vi "Get Measurements P2.vi"(0 "Image In":T1, 11 "Error In":errorcluster) -> (4 "Image Out":T1, 12 "Calibrated Results (P2 Hole)":sgl format="%.2f", 13 "Calibrated Results (P2 Right Edge Angle)":sgl, 14 "Calibrated Results (P2 Left Edge Angles)":sgl, 15 "Error Out":errorcluster)   [LabVIEW 2020]
uses:
  <vilib>/vision/Image Controls.llb/IMAQ Image.ctl
  <vilib>/vision/Measure.llb/Edge Options.ctl
  <vilib>/vision/Measure.llb/Edge Polarity.ctl
  <vilib>/vision/Measure.llb/Straight Edge Options.ctl
  <vilib>/vision/Measure.llb/Straight Edge Process.ctl
  <vilib>/vision/NI_Vision_Development_Module.lvlib
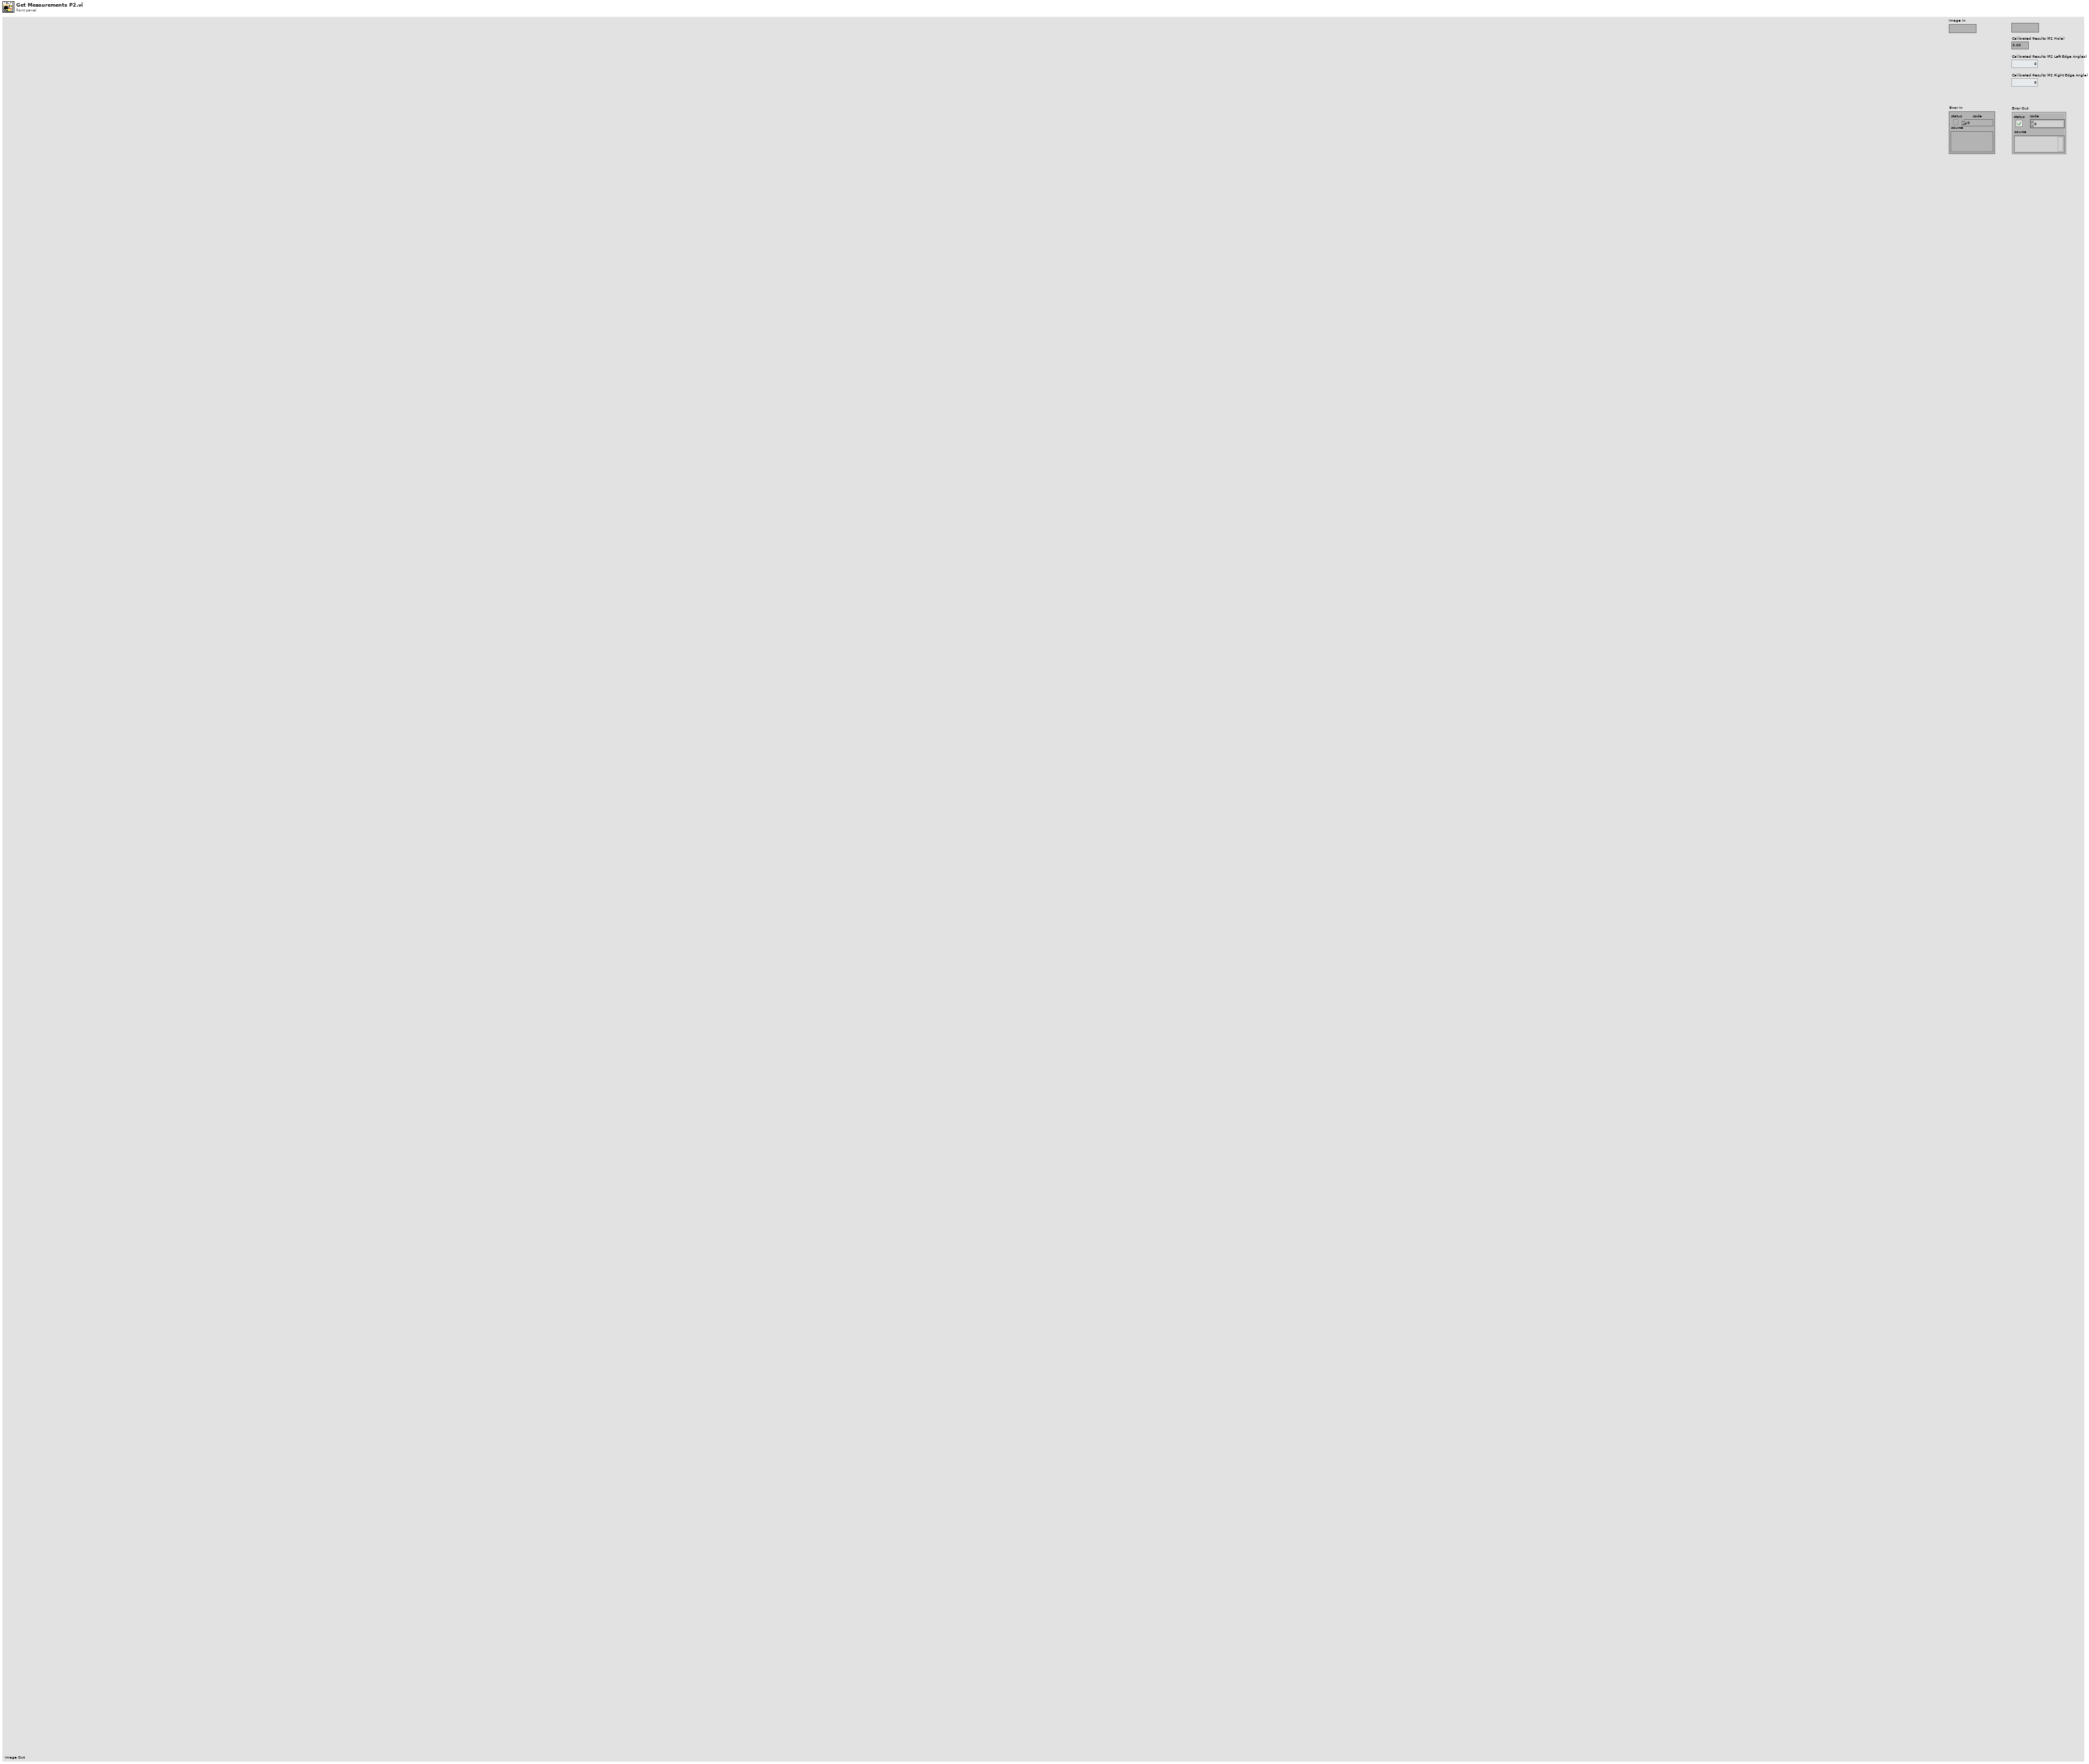
[diagram p1: front panel]
types:
  T1 = typedef "IMAQ Image.ctl" = refnum<image>
  T2 = cluster{"Feature":u32, "Points IDs":cluster{"GUID":string, "Index":i32}[]}[]
  T3 = typedef "Edge Options.ctl" = cluster{"Edge Polarity":T4, "Kernel Size":u32, "Width":u32, "Minimum Edge Strength":sgl, "Interpolation Type":enum32{"Zero Order", "Bilinear", "Quadratic", "Cubic", "Bilinear Fixed"}, "Data Processing Method":enum32{"Average", "Median"}}
  T4 = typedef "Edge Polarity.ctl" = u32
  T5 = cluster{"Search Direction":u32, "Edge Options":T3, "Show Search Area":bool, "Show Search Lines":bool, "Show Edges Found":bool, "Show Result":bool, "Search Area Color":u32, "Search Lines Color":u32, "Edge Locations Color":u32, "Result Color":u32, "Overlay Group Name":string}
  T6 = typedef "Straight Edge Options.ctl" = cluster{"Number of Lines":i32, "Type":T7, "Min. Score":dbl, "Max. Score":dbl, "Orientation":dbl, "Angle Range":dbl, "Angle Tolerance":dbl, "Step Size":u32, "Min. SNR (db)":dbl, "Min. Points (%)":dbl, "Hough Iterations":i32}
  T7 = typedef "Straight Edge Process.ctl" = enum32{"First Edge Rake", "Best Edge Rake", "Hough Edge Rake", "First Edge Projection", "Best Edge Projection"}
  T8 = cluster{"Global Rectangle":i32[], "Contours":cluster{"ID":enum32{"External", "Internal"}, "Type":u32, "Coordinates":i32[]}[]}
  T9 = cluster{"Origin":cluster{"X":sgl, "Y":sgl}, "Angle (deg)":sgl, "Axis Reference":u32}
  T10 = enum16{"Reset", "Update Coordinate System", "Get Coordinate System"}
  T11 = cluster{"Search  Direction":u32, "Edge Options":T3, "Show Search Area":bool, "Show Search Lines":bool, "Show Edges Found":bool, "Show Result":bool, "Search Area Color":u32, "Search Lines Color":u32, "Edge Locations Color":u32, "Result Color":u32, "Overlay Group Name":string}
  T12 = cluster{"Process":enum16{"Get First Edge", "Get First + Last Edge", "Get All Edges", "Get Best Edge"}, "Step Size":i32, "Max Pixel Radius":i32}
  T13 = typedef "IMAQ Coordinate System" = cluster{"Reference System":cluster{"Origin":cluster{"X":sgl, "Y":sgl}, "Angle (deg)":sgl, "Axis Reference":u32}, "Measurement System":cluster{"Origin":cluster{"X":sgl, "Y":sgl}, "Angle (deg)":sgl, "Axis Reference":u32}}
  T14 = typedef "ROI Descriptor" = cluster{"Global Rectangle":i32[], "Contours":cluster{"ID":enum32{"External", "Internal"}, "Type":u32, "Coordinates":i32[]}[]}
  T15 = cluster{"Point1 (Pixels)":cluster{"X":sgl, "Y":sgl}, "Point2 (Pixels)":cluster{"X":sgl, "Y":sgl}, "Point1 (Real-World)":cluster{"X":sgl, "Y":sgl}, "Point2 (Real-World)":cluster{"X":sgl, "Y":sgl}, "Angle (Pixel)":dbl, "Angle (Real-World)":dbl, "Score":dbl, "Straightness":dbl, "Average SNR (db)":dbl, "Calibration Valid":bool}[]
  T16 = cluster{"Point1 (Pixels)":cluster{"X":sgl, "Y":sgl}, "Point2 (Pixels)":cluster{"X":sgl, "Y":sgl}, "Point1 (Real-World)":cluster{"X":sgl, "Y":sgl}, "Point2 (Real-World)":cluster{"X":sgl, "Y":sgl}, "Angle (Pixel)":dbl, "Angle (Real-World)":dbl, "Score":dbl, "Straightness":dbl, "Average SNR (db)":dbl, "Calibration Valid":bool}
  T17 = cluster{"Center (Pixels)":cluster{"X":sgl, "Y":sgl}, "Radius (Pixels)":dbl, "Center (Real-World)":cluster{"X":sgl, "Y":sgl}, "Radius (Real-World)":dbl, "Roundness (Real-World)":dbl, "Average Strength":dbl, "Average SNR (dB)":dbl}
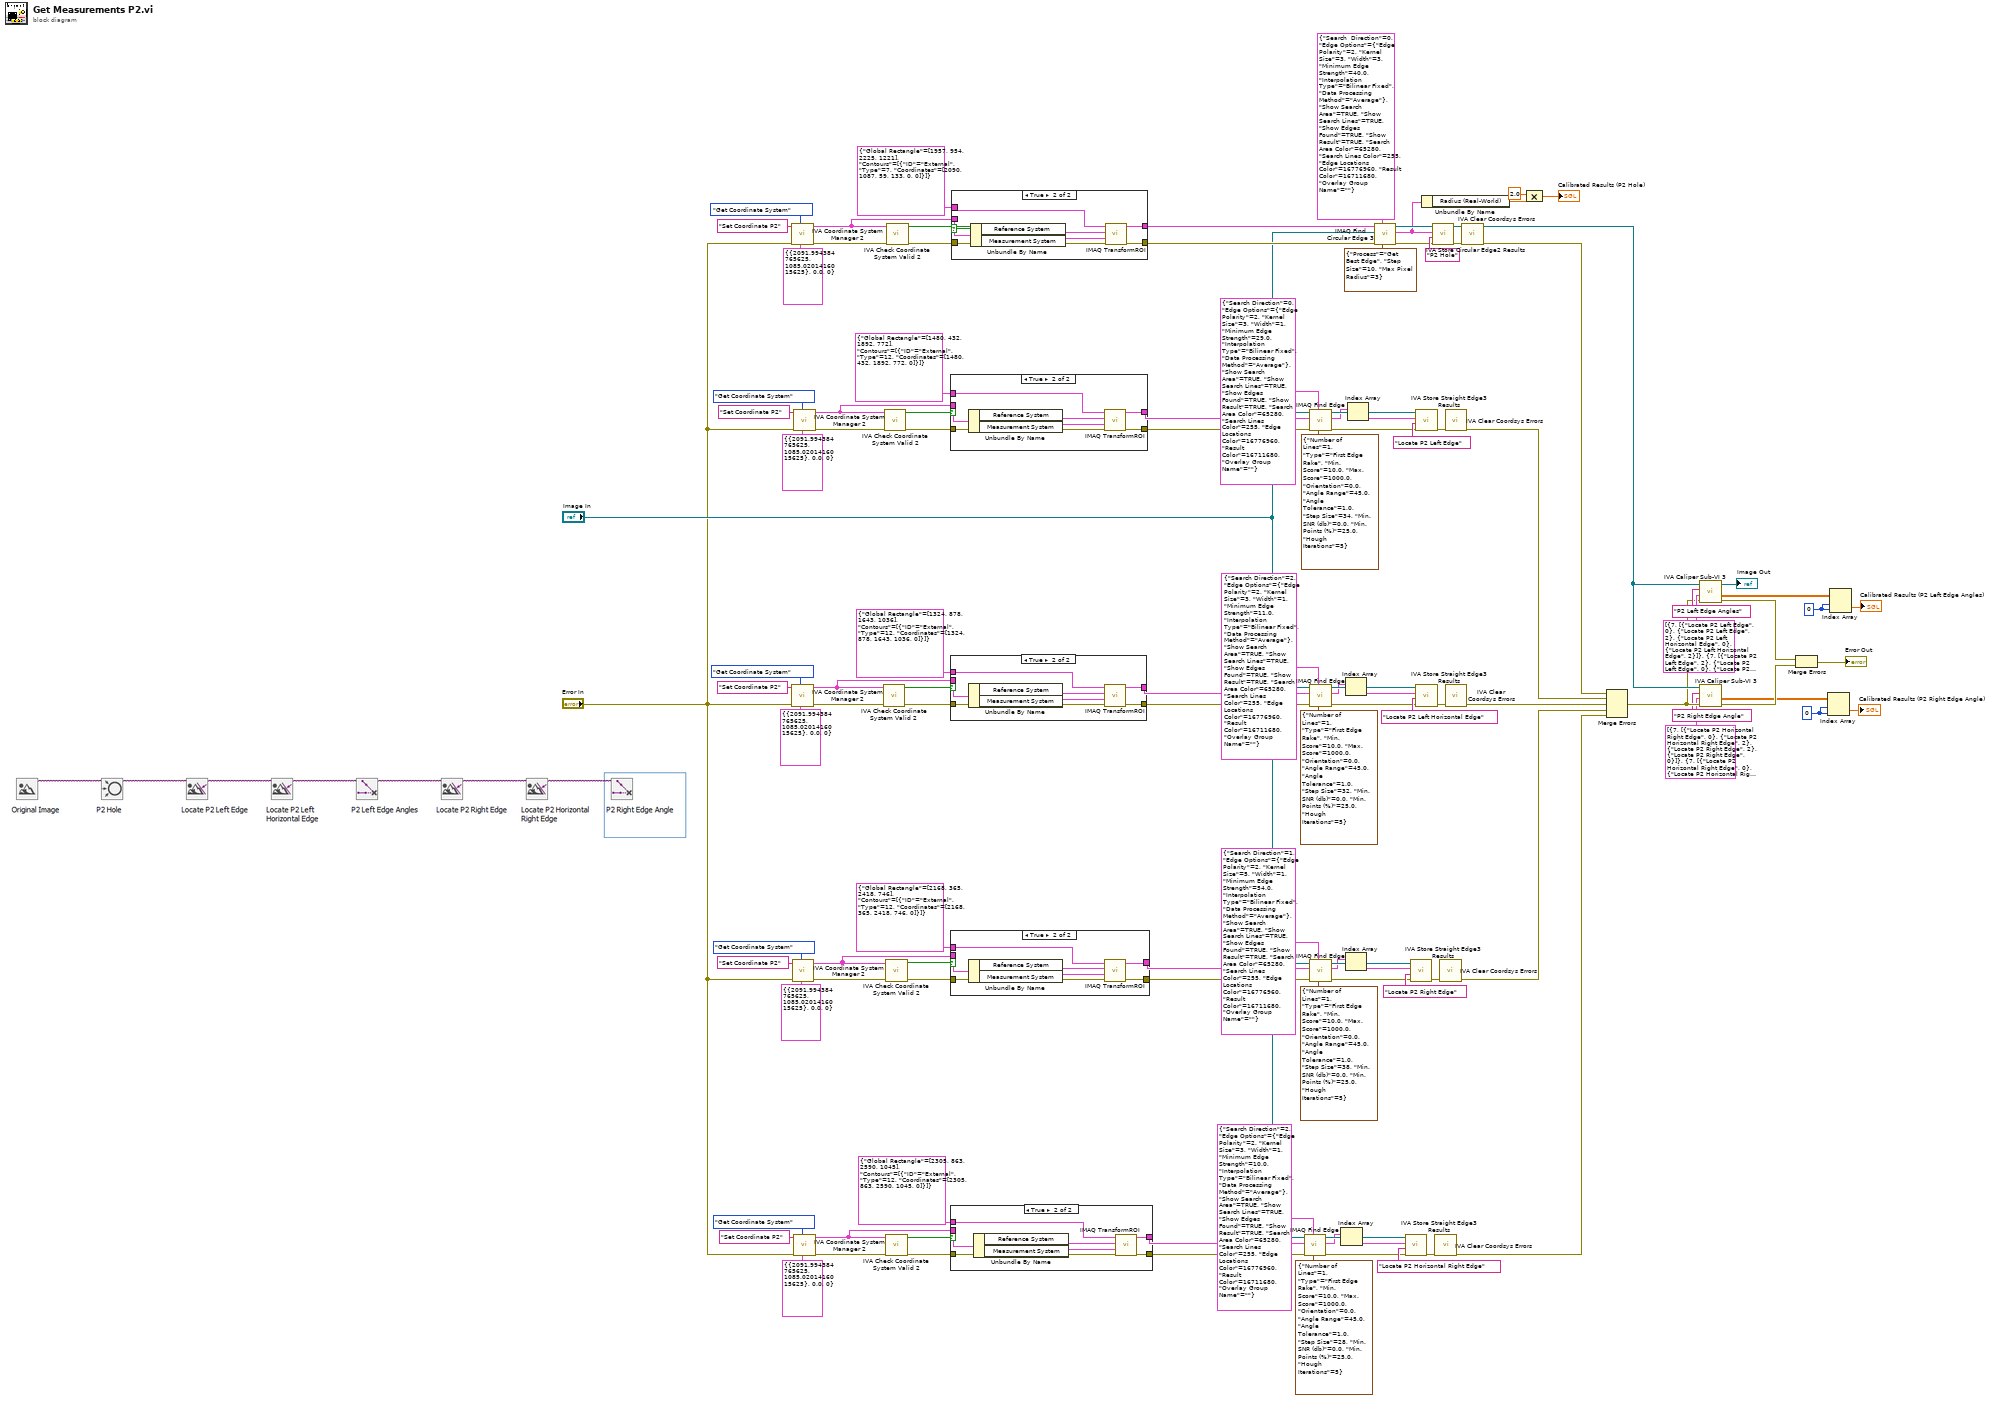
[diagram p0: block diagram]
diagram:
  w5 = 0 ("disabled index (col)")
  w6 = 0 ("disabled index (col)")
  n1 = call <vilib>:"IVA Coordinate System Manager 2.vi"("Reference System"=T9 {"Origin"={"X"=2091.9944, "Y"=1085.0201}, "Angle (deg)"=0.0, "Axis Reference"=0}, "Function"=T10."Get Coordinate System", "error in (no error)"="Error In", "Coordinate System Name"="Set Coordinate P2") -> ("error out"=w109:errorcluster, "Coordinate System Out"=w111:T13)  [unwired: 3 in, 3 out]
  n2 = call <vilib>:"IVA Coordinate System Manager 2.vi"("Reference System"=T9 {"Origin"={"X"=2091.9944, "Y"=1085.0201}, "Angle (deg)"=0.0, "Axis Reference"=0}, "Function"=T10."Get Coordinate System", "error in (no error)"="Error In", "Coordinate System Name"="Set Coordinate P2") -> ("error out"=w75:errorcluster, "Coordinate System Out"=w77:T13)  [unwired: 3 in, 3 out]
  n3 = call <vilib>:"IVA Coordinate System Manager 2.vi"("Reference System"=T9 {"Origin"={"X"=2091.9944, "Y"=1085.0201}, "Angle (deg)"=0.0, "Axis Reference"=0}, "Function"=T10."Get Coordinate System", "error in (no error)"="Error In", "Coordinate System Name"="Set Coordinate P2") -> ("error out"=w57:errorcluster, "Coordinate System Out"=w59:T13)  [unwired: 3 in, 3 out]
  n4 = call <vilib>:"IVA Coordinate System Manager 2.vi"("Reference System"=T9 {"Origin"={"X"=2091.9944, "Y"=1085.0201}, "Angle (deg)"=0.0, "Axis Reference"=0}, "Function"=T10."Get Coordinate System", "error in (no error)"="Error In", "Coordinate System Name"="Set Coordinate P2") -> ("error out"=w93:errorcluster, "Coordinate System Out"=w95:T13)  [unwired: 3 in, 3 out]
  n5 = call <vilib>:"IVA Coordinate System Manager 2.vi"("Reference System"=T9 {"Origin"={"X"=2091.9944, "Y"=1085.0201}, "Angle (deg)"=0.0, "Axis Reference"=0}, "Function"=T10."Get Coordinate System", "error in (no error)"="Error In", "Coordinate System Name"="Set Coordinate P2") -> ("error out"=w39:errorcluster, "Coordinate System Out"=w41:T13)  [unwired: 3 in, 3 out]
  n6 = call <vilib>:"IVA Check Coordinate System Valid 2.vi"("error in (no error)"=w75, "Coordinate System"=w77) -> ("error out"=w74:errorcluster, "Valid?"=w76:bool)  [unwired: 8 out]
  n7 = call <vilib>:"IVA Check Coordinate System Valid 2.vi"("error in (no error)"=w93, "Coordinate System"=w95) -> ("error out"=w92:errorcluster, "Valid?"=w94:bool)  [unwired: 8 out]
  n8 = call <vilib>:"IVA Check Coordinate System Valid 2.vi"("error in (no error)"=w57, "Coordinate System"=w59) -> ("error out"=w56:errorcluster, "Valid?"=w58:bool)  [unwired: 8 out]
  n9 = call <vilib>:"IVA Check Coordinate System Valid 2.vi"("error in (no error)"=w39, "Coordinate System"=w41) -> ("error out"=w38:errorcluster, "Valid?"=w40:bool)  [unwired: 8 out]
  n10 = call <vilib>:"IVA Check Coordinate System Valid 2.vi"("error in (no error)"=w109, "Coordinate System"=w111) -> ("error out"=w108:errorcluster, "Valid?"=w110:bool)  [unwired: 8 out]
  n11 = case shown="True" w94 {
    tunnel: T8 {"Global Rectangle"=[1480, 432, 1892, 772], "Contours"=[{"ID"=enum."External", "Type"=12, "Coordinates"=[1480, 432, 1892, 772, 0]}]} ("ROI Descriptor") -> [w117 w124]
    tunnel: [w117 w121] -> w91
    tunnel: [w116 w120] -> w89
    tunnel: w95 -> [_ w119]
    tunnel: w92 -> [w116 w118]
    frame False {
    }
    frame True {
      n12 = Unbundle By Name(w119) -> ("Reference System"=w123:T9, "Measurement System"=w122:T9)
      n13 = call "IMAQ TransformROI"("error in (no error)"=w118, "New Reference"=w122, "Base Reference"=w123, "ROI Descriptor"=w124) -> ("error out"=w120:errorcluster, "ROI Descriptor out"=w121:T14)  [unwired: 6 out]
    }
  }
  n14 = case shown="True" w76 {
    tunnel: T8 {"Global Rectangle"=[1324, 878, 1643, 1036], "Contours"=[{"ID"=enum."External", "Type"=12, "Coordinates"=[1324, 878, 1643, 1036, 0]}]} ("ROI Descriptor") -> [w126 w133]
    tunnel: [w126 w130] -> w73
    tunnel: [w125 w129] -> w71
    tunnel: w77 -> [_ w128]
    tunnel: w74 -> [w125 w127]
    frame False {
    }
    frame True {
      n15 = Unbundle By Name(w128) -> ("Reference System"=w132:T9, "Measurement System"=w131:T9)
      n16 = call "IMAQ TransformROI"("error in (no error)"=w127, "New Reference"=w131, "Base Reference"=w132, "ROI Descriptor"=w133) -> ("error out"=w129:errorcluster, "ROI Descriptor out"=w130:T14)  [unwired: 6 out]
    }
  }
  n17 = case shown="True" w58 {
    tunnel: T8 {"Global Rectangle"=[2168, 365, 2418, 746], "Contours"=[{"ID"=enum."External", "Type"=12, "Coordinates"=[2168, 365, 2418, 746, 0]}]} ("ROI Descriptor") -> [w135 w142]
    tunnel: [w135 w139] -> w55
    tunnel: [w134 w138] -> w53
    tunnel: w59 -> [_ w137]
    tunnel: w56 -> [w134 w136]
    frame False {
    }
    frame True {
      n18 = Unbundle By Name(w137) -> ("Reference System"=w141:T9, "Measurement System"=w140:T9)
      n19 = call "IMAQ TransformROI"("error in (no error)"=w136, "New Reference"=w140, "Base Reference"=w141, "ROI Descriptor"=w142) -> ("error out"=w138:errorcluster, "ROI Descriptor out"=w139:T14)  [unwired: 6 out]
    }
  }
  n20 = case shown="True" w40 {
    tunnel: T8 {"Global Rectangle"=[2305, 863, 2590, 1045], "Contours"=[{"ID"=enum."External", "Type"=12, "Coordinates"=[2305, 863, 2590, 1045, 0]}]} ("ROI Descriptor") -> [w144 w151]
    tunnel: [w144 w148] -> w37
    tunnel: [w143 w147] -> w35
    tunnel: w41 -> [_ w146]
    tunnel: w38 -> [w143 w145]
    frame False {
    }
    frame True {
      n21 = Unbundle By Name(w146) -> ("Reference System"=w150:T9, "Measurement System"=w149:T9)
      n22 = call "IMAQ TransformROI"("error in (no error)"=w145, "New Reference"=w149, "Base Reference"=w150, "ROI Descriptor"=w151) -> ("error out"=w147:errorcluster, "ROI Descriptor out"=w148:T14)  [unwired: 6 out]
    }
  }
  n23 = case shown="True" w110 {
    tunnel: T8 {"Global Rectangle"=[1957, 954, 2225, 1221], "Contours"=[{"ID"=enum."External", "Type"=7, "Coordinates"=[2090, 1087, 59, 133, 0, 0]}]} ("ROI Descriptor") -> [w153 w160]
    tunnel: [w153 w157] -> w106
    tunnel: [w152 w156] -> w105
    tunnel: w111 -> [_ w155]
    tunnel: w108 -> [w152 w154]
    frame False {
    }
    frame True {
      n24 = Unbundle By Name(w155) -> ("Reference System"=w159:T9, "Measurement System"=w158:T9)
      n25 = call "IMAQ TransformROI"("error in (no error)"=w154, "New Reference"=w158, "Base Reference"=w159, "ROI Descriptor"=w160) -> ("error out"=w156:errorcluster, "ROI Descriptor out"=w157:T14)  [unwired: 6 out]
    }
  }
  n26 = call "IMAQ Find Edge"("Line Fit Options"=T6 {"Number of Lines"=1, "Type"=enum."First Edge Rake", "Min. Score"=10.0, "Max. Score"=1000.0, "Orientation"=0.0, "Angle Range"=45.0, "Angle Tolerance"=1.0, "Step Size"=28, "Min. SNR (db)"=0.0, "Min. Points (%)"=25.0, "Hough Iterations"=5} ("Fit Options"), "Options"=T5 {"Search Direction"=2, "Edge Options"={"Edge Polarity"=2, "Kernel Size"=3, "Width"=1, "Minimum Edge Strength"=10.0, "Interpolation Type"=enum."Bilinear Fixed", "Data Processing Method"=enum."Average"}, "Show Search Area"=TRUE, "Show Search Lines"=TRUE, "Show Edges Found"=TRUE, "Show Result"=TRUE, "Search Area Color"=65280, "Search Lines Color"=255, "Edge Locations Color"=16776960, "Result Color"=16711680, "Overlay Group Name"=""}, "error in (no error)"=w35, "ROI Descriptor"=w37, "Image"="Image In") -> ("error out"=w30:errorcluster, "Straight Edges"=w29:T15, "Image Out"=w31:T1)  [unwired: 1 in, 3 out]
  n27 = call "IMAQ Find Edge"("Line Fit Options"=T6 {"Number of Lines"=1, "Type"=enum."First Edge Rake", "Min. Score"=10.0, "Max. Score"=1000.0, "Orientation"=0.0, "Angle Range"=45.0, "Angle Tolerance"=1.0, "Step Size"=34, "Min. SNR (db)"=0.0, "Min. Points (%)"=25.0, "Hough Iterations"=5} ("Fit Options"), "Options"=T5 {"Search Direction"=0, "Edge Options"={"Edge Polarity"=2, "Kernel Size"=3, "Width"=1, "Minimum Edge Strength"=29.0, "Interpolation Type"=enum."Bilinear Fixed", "Data Processing Method"=enum."Average"}, "Show Search Area"=TRUE, "Show Search Lines"=TRUE, "Show Edges Found"=TRUE, "Show Result"=TRUE, "Search Area Color"=65280, "Search Lines Color"=255, "Edge Locations Color"=16776960, "Result Color"=16711680, "Overlay Group Name"=""}, "error in (no error)"=w89, "ROI Descriptor"=w91, "Image"="Image In") -> ("error out"=w84:errorcluster, "Straight Edges"=w83:T15, "Image Out"=w85:T1)  [unwired: 1 in, 3 out]
  n28 = call "IMAQ Find Edge"("Line Fit Options"=T6 {"Number of Lines"=1, "Type"=enum."First Edge Rake", "Min. Score"=10.0, "Max. Score"=1000.0, "Orientation"=0.0, "Angle Range"=45.0, "Angle Tolerance"=1.0, "Step Size"=32, "Min. SNR (db)"=0.0, "Min. Points (%)"=25.0, "Hough Iterations"=5} ("Fit Options"), "Options"=T5 {"Search Direction"=2, "Edge Options"={"Edge Polarity"=2, "Kernel Size"=3, "Width"=1, "Minimum Edge Strength"=11.0, "Interpolation Type"=enum."Bilinear Fixed", "Data Processing Method"=enum."Average"}, "Show Search Area"=TRUE, "Show Search Lines"=TRUE, "Show Edges Found"=TRUE, "Show Result"=TRUE, "Search Area Color"=65280, "Search Lines Color"=255, "Edge Locations Color"=16776960, "Result Color"=16711680, "Overlay Group Name"=""}, "error in (no error)"=w71, "ROI Descriptor"=w73, "Image"="Image In") -> ("error out"=w66:errorcluster, "Straight Edges"=w65:T15, "Image Out"=w67:T1)  [unwired: 1 in, 3 out]
  n29 = call "IMAQ Find Edge"("Line Fit Options"=T6 {"Number of Lines"=1, "Type"=enum."First Edge Rake", "Min. Score"=10.0, "Max. Score"=1000.0, "Orientation"=0.0, "Angle Range"=45.0, "Angle Tolerance"=1.0, "Step Size"=38, "Min. SNR (db)"=0.0, "Min. Points (%)"=25.0, "Hough Iterations"=5} ("Fit Options"), "Options"=T5 {"Search Direction"=1, "Edge Options"={"Edge Polarity"=2, "Kernel Size"=5, "Width"=1, "Minimum Edge Strength"=54.0, "Interpolation Type"=enum."Bilinear Fixed", "Data Processing Method"=enum."Average"}, "Show Search Area"=TRUE, "Show Search Lines"=TRUE, "Show Edges Found"=TRUE, "Show Result"=TRUE, "Search Area Color"=65280, "Search Lines Color"=255, "Edge Locations Color"=16776960, "Result Color"=16711680, "Overlay Group Name"=""}, "error in (no error)"=w53, "ROI Descriptor"=w55, "Image"="Image In") -> ("error out"=w48:errorcluster, "Straight Edges"=w47:T15, "Image Out"=w49:T1)  [unwired: 1 in, 3 out]
  n30 = Index Array(array=w29) -> (element=w32:T16)  [unwired: 1 in]
  n31 = Index Array(array=w65) -> (element=w68:T16)  [unwired: 1 in]
  n32 = Index Array(array=w47) -> (element=w50:T16)  [unwired: 1 in]
  n33 = Index Array(array=w83) -> (element=w86:T16)  [unwired: 1 in]
  n34 = call "IMAQ Find Circular Edge 3"("Circle Fit Options"=T12 {"Process"=enum."Get Best Edge", "Step Size"=10, "Max Pixel Radius"=3}, "Options"=T11 {"Search  Direction"=0, "Edge Options"={"Edge Polarity"=2, "Kernel Size"=3, "Width"=3, "Minimum Edge Strength"=40.0, "Interpolation Type"=enum."Bilinear Fixed", "Data Processing Method"=enum."Average"}, "Show Search Area"=TRUE, "Show Search Lines"=TRUE, "Show Edges Found"=TRUE, "Show Result"=TRUE, "Search Area Color"=65280, "Search Lines Color"=255, "Edge Locations Color"=16776960, "Result Color"=16711680, "Overlay Group Name"=""}, "error in (no error)"=w105, "ROI Descriptor"=w106, "Image"="Image In") -> ("error out"=w102:errorcluster, "Fitted Circle"=w12:T17, "Image Out"=w101:T1)  [unwired: 2 in, 2 out]
  n35 = call <vilib>:"IVA Store Straight Edge3 Results.vi"("error in (no error)"=w30, "Step Name"="Locate P2 Horizontal Right Edge", "Straight Edge"=w32, "Image in"=w31) -> ("error out"=w28:errorcluster)  [unwired: 1 in, 6 out]
  n36 = call <vilib>:"IVA Store Straight Edge3 Results.vi"("error in (no error)"=w48, "Step Name"="Locate P2 Right Edge", "Straight Edge"=w50, "Image in"=w49) -> ("error out"=w46:errorcluster)  [unwired: 1 in, 6 out]
  n37 = call <vilib>:"IVA Store Straight Edge3 Results.vi"("error in (no error)"=w84, "Step Name"="Locate P2 Left Edge", "Straight Edge"=w86, "Image in"=w85) -> ("error out"=w82:errorcluster)  [unwired: 1 in, 6 out]
  n38 = call <vilib>:"IVA Store Straight Edge3 Results.vi"("error in (no error)"=w66, "Step Name"="Locate P2 Left Horizontal Edge", "Straight Edge"=w68, "Image in"=w67) -> ("error out"=w64:errorcluster)  [unwired: 1 in, 6 out]
  n39 = Unbundle By Name(w12) -> ("Radius (Real-World)"=w11:dbl)
  n40 = call <vilib>:"IVA Store Circular Edge2 Results.vi"("error in (no error)"=w102, "Step Name"="P2 Hole", "Fitted Circle"=w12, "Image in"=w101) -> ("error out"=w100:errorcluster, "Image dup"=w20:T1)  [unwired: 2 in, 4 out]
  n41 = call <vilib>:"IVA Clear Coordsys Errors.vi"("error in (no error)"=w28) -> ("error out"=w23:errorcluster)  [unwired: 10 in]
  n42 = call <vilib>:"IVA Clear Coordsys Errors.vi"("error in (no error)"=w46) -> ("error out"=w24:errorcluster)  [unwired: 10 in]
  n43 = call <vilib>:"IVA Clear Coordsys Errors.vi"("error in (no error)"=w82) -> ("error out"=w26:errorcluster)  [unwired: 10 in]
  n44 = call <vilib>:"IVA Clear Coordsys Errors.vi"("error in (no error)"=w64) -> ("error out"=w25:errorcluster)  [unwired: 10 in]
  n45 = call <vilib>:"IVA Clear Coordsys Errors.vi"("error in (no error)"=w100) -> ("error out"=w27:errorcluster)  [unwired: 10 in]
  n46 = Compound Arithmetic op=MULTIPLY(2.0 ("value"), w11) -> (→"Calibrated Results (P2 Hole)":dbl)
  n47 = Merge Errors(w27, w26, w25, w24, w23) -> (w19:errorcluster)
  n48 = call <vilib>:"IVA Caliper Sub-VI 3.vi"("error in"=w19, "Parameters"=T2 [{"Feature"=7, "Points IDs"=[{"GUID"="Locate P2 Left Edge", "Index"=0}, {"GUID"="Locate P2 Left Edge", "Index"=2}, {"GUID"="Locate P2 Left Horizontal Edge", "Index"=0}, {"GUID"="Locate P2 Left Horizontal Edge", "Index"=2}]}, {"Feature"=7, "Points IDs"=[{"GUID"="Locate P2 Left Edge", "Index"=2}, {"GUID"="Locate P2 Left Edge", "Index"=0}, {"GUID"="Locate P2 Left Horizontal Edge", "Index"=2}, {"GUID"="Locate P2 Left Horizontal Edge", "Index"=0}]}, {"Feature"=7, "Points IDs"=[{"GUID"="Locate P2 Left Edge", "Index"=0}, {"GUID"="Locate P2 Left Edge", "Index"=2}, {"GUID"="Locate P2 Left Horizontal Edge", "Index"=0}, {"GUID"="Locate P2 Left Horizontal Edge", "Index"=2}]}], "Step Name"="P2 Left Edge Angles", "Image In"=w20) -> ("error out"=w14:errorcluster, "Results (Calibrated)"=w8:sgl[][], "Image Out"=→"Image Out":T1)  [unwired: 1 in, 4 out]
  n49 = call <vilib>:"IVA Caliper Sub-VI 3.vi"("error in"=w19, "Parameters"=T2 [{"Feature"=7, "Points IDs"=[{"GUID"="Locate P2 Horizontal Right Edge", "Index"=0}, {"GUID"="Locate P2 Horizontal Right Edge", "Index"=2}, {"GUID"="Locate P2 Right Edge", "Index"=2}, {"GUID"="Locate P2 Right Edge", "Index"=0}]}, {"Feature"=7, "Points IDs"=[{"GUID"="Locate P2 Horizontal Right Edge", "Index"=0}, {"GUID"="Locate P2 Horizontal Right Edge", "Index"=2}, {"GUID"="Locate P2 Right Edge", "Index"=2}, {"GUID"="Locate P2 Right Edge", "Index"=0}]}, {"Feature"=7, "Points IDs"=[{"GUID"="Locate P2 Horizontal Right Edge", "Index"=0}, {"GUID"="Locate P2 Horizontal Right Edge", "Index"=2}, {"GUID"="Locate P2 Right Edge", "Index"=2}, {"GUID"="Locate P2 Right Edge", "Index"=0}]}, {"Feature"=7, "Points IDs"=[{"GUID"="Locate P2 Horizontal Right Edge", "Index"=0}, {"GUID"="Locate P2 Horizontal Right Edge", "Index"=2}, {"GUID"="Locate P2 Right Edge", "Index"=2}, {"GUID"="Locate P2 Right Edge", "Index"=0}]}, {"Feature"=7, "Points IDs"=[{"GUID"="Locate P2 Horizontal Right Edge", "Index"=0}, {"GUID"="Locate P2 Horizontal Right Edge", "Index"=2}, {"GUID"="Locate P2 Right Edge", "Index"=2}, {"GUID"="Locate P2 Right Edge", "Index"=0}]}, {"Feature"=7, "Points IDs"=[{"GUID"="Locate P2 Horizontal Right Edge", "Index"=0}, {"GUID"="Locate P2 Horizontal Right Edge", "Index"=2}, {"GUID"="Locate P2 Right Edge", "Index"=2}, {"GUID"="Locate P2 Right Edge", "Index"=0}]}, {"Feature"=7, "Points IDs"=[{"GUID"="Locate P2 Horizontal Right Edge", "Index"=0}, {"GUID"="Locate P2 Horizontal Right Edge", "Index"=2}, {"GUID"="Locate P2 Right Edge", "Index"=2}, {"GUID"="Locate P2 Right Edge", "Index"=0}]}, {"Feature"=7, "Points IDs"=[{"GUID"="Locate P2 Horizontal Right Edge", "Index"=0}, {"GUID"="Locate P2 Horizontal Right Edge", "Index"=2}, {"GUID"="Locate P2 Right Edge", "Index"=2}, {"GUID"="Locate P2 Right Edge", "Index"=0}]}], "Step Name"="P2 Right Edge Angle", "Image In"=w20) -> ("error out"=w15:errorcluster, "Results (Calibrated)"=w4:sgl[][])  [unwired: 1 in, 5 out]
  n50 = Merge Errors(w14, w15) -> (→"Error Out":errorcluster)
  n51 = Index Array(array=w4, index (row)=w5, index (col)=w5) -> (element=→"Calibrated Results (P2 Right Edge Angle)":sgl)
  n52 = Index Array(array=w8, index (row)=w6, index (col)=w6) -> (element=→"Calibrated Results (P2 Left Edge Angles)":sgl)
